vi "Convert Pump RPMs.vi"(11 "RPMs input":i64[](array[numeric])) -> (3 "RPMs Output":i64[](array[numeric]))   [LabVIEW 2024, in "UI.lvlib"]
uses:
  UI.lvlib
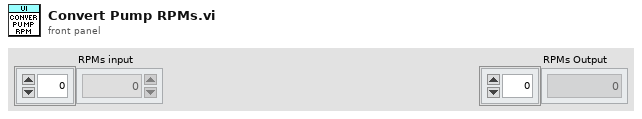
[diagram p1: front panel]
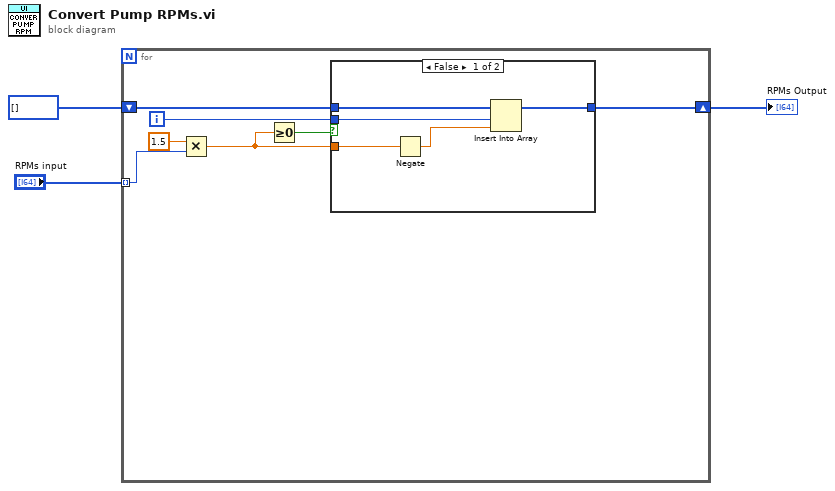
[diagram p0: block diagram]
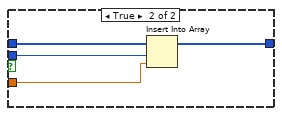
[diagram p2: hidden frame]
diagram:
  n1 = for {
    shift-right: [w9] -> w2
    shift-left: i64[] [] ("RPMs Output") -> [w10]
    tunnel: "RPMs input" -> [w7] mode=indexing
    i -> [w8]
    n2 = Multiply(x=1.5, y=w7) -> (x*y=w5:dbl)
    n3 = Greater Or Equal To 0?(x=w5) -> (x >= 0?=w4:bool)
    n4 = case shown="False" w4 {
      tunnel: w10 -> [w14 w19]
      tunnel: [w15 w18] -> w9
      tunnel: w8 -> [w13 w17]
      tunnel: w5 -> [w12 w16]
      frame False {
        n5 = Negate(x=w12) -> (-x=w11:dbl)
        n6 = Insert Into Array(array=w14, index=w13, new element=w11) -> (w15:i64[])
      }
      frame True {
        n7 = Insert Into Array(array=w19, index=w17, new element=w16) -> (w18:i64[])
      }
    }
  }
  "RPMs Output" <- w2
